vi "ask_test.vi"() -> ()   [LabVIEW 2012]
uses:
  <vilib>/addons/Modulation/Digital/General/MT Generate ASK system parameters (M).vi
  <vilib>/addons/Modulation/Digital/General/MT Generate ASK Synchronization Parameters (bit array).vi
  <vilib>/addons/Modulation/niDMT.lvlib
panel:
  out "Waveform Graph 2":dbl[](graph)
  out "Waveform Graph":dbl[](graph)
  out "ber":dbl
  out "error out":errorcluster
  out "output bit stream":i8[](array[numeric])
  out "appended array":i8[](array[numeric])
  out "Key Bit Sequence":i8[](array[numeric])
  in  "Packet Length":i32
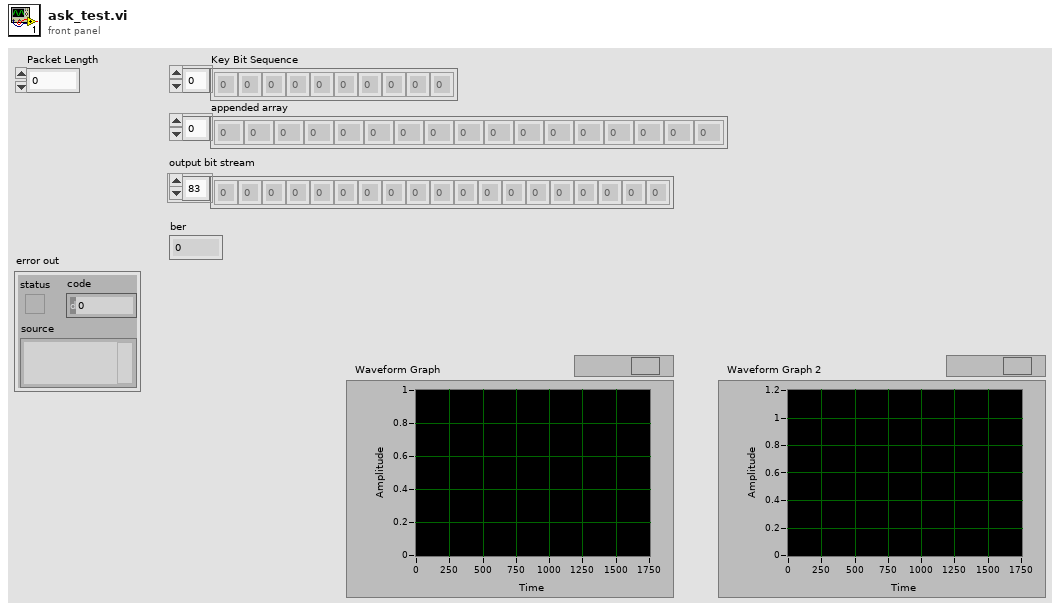
[diagram p1: front panel]
types:
  T1 = enum16{"FSK", "PSK", "QAM", "MSK", "PAM", "ASK", "CPM"}
  T2 = cluster{"samples per symbol (16)":i32, "symbol map":cdb[]}
  T3 = typedef "niAMT.lvlib/Complex Data Waveform.ctl" = cluster{"t0":dbl, "dt":dbl, "Y":cdb[]}
  T4 = cluster{"expected sync location (symbols)":i32, "sync sequence":cdb[], "sync location uncertainty (symbols)":i32, "sync indent (symbols)":i32}
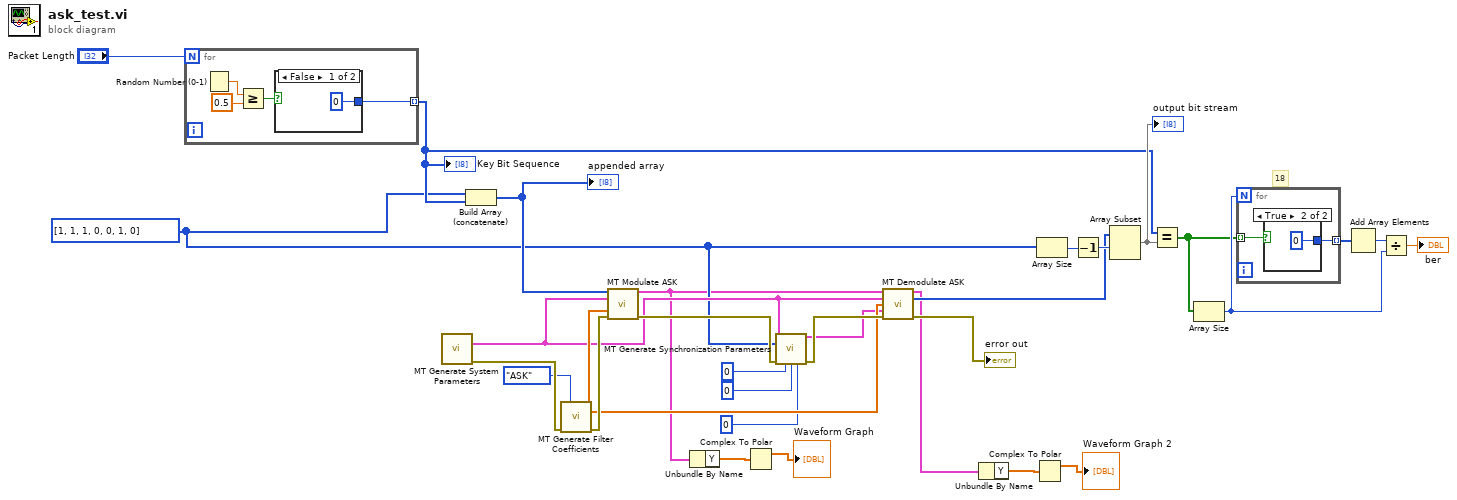
[diagram p0: block diagram]
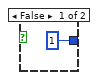
[diagram p2: hidden frame]
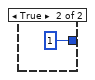
[diagram p3: hidden frame]
diagram:
  w10 = i8[] [1, 1, 1, 0, 0, 1, 0] ("sync bits")
  # "18"
  n1 = for {
    N: "Packet Length" -> [_]
    tunnel: [w33] -> w13 mode=indexing
    n2 = Random Number (0-1)() -> (number: 0 to 1=w35:dbl)
    n3 = Greater Or Equal?(x=w35, y=0.5) -> (x >= y?=w34:bool)
    n4 = case shown="False" w34 {
      tunnel: [i8 0 i8 1] -> w33
      frame False {
      }
      frame True {
      }
    }
  }
  "Key Bit Sequence" <- w13
  n5 = call-poly <vilib>:"MT Generate System Parameters.vi"() -> ("ASK system parameters"=w24:T2, "error out"=w32:errorcluster)  [unwired: 13 in, 1 out]
  n6 = Build Array (concatenate)(w10, w13) -> (w22:i8[])
  "appended array" <- w22
  n7 = call <vilib>:"MT Generate Filter Coefficients.vi"("modulation type"=T1."ASK", "error in (no error)"=w32) -> ("pulse shaping filter coefficients"=w28:dbl[], "matched filter coefficients"=w27:dbl[], "error out"=w31:errorcluster)  [unwired: 11 in]
  n8 = call <vilib>:"MT Modulate ASK.vi"("input bit stream"=w22, "ASK system parameters"=w24, "pulse shaping filter coefficients"=w28, "error in (no error)"=w31) -> ("output complex waveform"=w9:T3, "error out"=w30:errorcluster)  [unwired: 9 in, 1 out]
  n9 = Unbundle By Name(w9) -> ("Y"=w8:cdb[])
  n10 = Complex To Polar(r * e^(i*theta)=w8) -> (r=→"Waveform Graph":dbl[])  [unwired: 1 out]
  n11 = call-poly <vilib>:"MT Generate Synchronization Parameters.vi"("ASK system parameters"=w24, "sync bits"=w10, "error in (no error)"=w30, "expected sync location (symbols)"=0, "sync location uncertainty (symbols)"=0 ("expected sync location (symbols)"), "sync indent (symbols)"=0) -> ("ASK synchronization parameters"=w26:T4, "error out"=w29:errorcluster)  [unwired: 8 in]
  n12 = call <vilib>:"MT Demodulate ASK.vi"("input complex waveform"=w9, "ASK system parameters"=w24, "matched filter coefficients"=w27, "synchronization parameters"=w26, "error in (no error)"=w29) -> ("recovered complex waveform"=w4:T3, "output bit stream"=w11:i8[], "error out"=→"error out":errorcluster)  [unwired: 6 in, 2 out]
  n13 = Unbundle By Name(w4) -> ("Y"=w6:cdb[])
  n14 = Complex To Polar(r * e^(i*theta)=w6) -> (r=→"Waveform Graph 2":dbl[])  [unwired: 1 out]
  n15 = Array Size(array=w10) -> (size(s)=w15:i32)
  n16 = Decrement(x=w15) -> (x-1=w14:i32)
  n17 = Array Subset(array=w11, index=w14) -> (w16:i8[])  [unwired: 1 in]
  "output bit stream" <- w16
  n18 = Equal?(x=w13, y=w16) -> (x = y?=w17:bool[])
  n19 = Array Size(array=w17) -> (size(s)=w19:i32)
  n20 = for {
    N: w19 -> [_]
    tunnel: [w40] -> w21 mode=indexing
    tunnel: w17 -> [w39] mode=indexing
    n21 = case shown="True" w39 {
      tunnel: [1 0] -> w40
      frame False {
      }
      frame True {
      }
    }
  }
  n22 = Add Array Elements(numeric array=w21) -> (sum=w20:i32)
  n23 = Divide(x=w20, y=w19) -> (x/y=→"ber":dbl)
